vi "Read outside terminal.vi"(9 "FlatSequenceInnerTunnel in":refnum<class "FlatSequenceOuterTunnel.lvclass">) -> (3 "FlatSequenceInnerTunnel out":refnum<class "FlatSequenceOuterTunnel.lvclass">, 4 "outside terminal":refnum<class "Terminal.lvclass">)   [LabVIEW 2014, in "FlatSequenceOuterTunnel.lvclass"]
uses:
  FlatSequenceOuterTunnel.lvclass
  Terminal/Terminal.lvclass
  FlatSequenceOuterTunnel.lvclass/FlatSequenceOuterTunnel.ctl
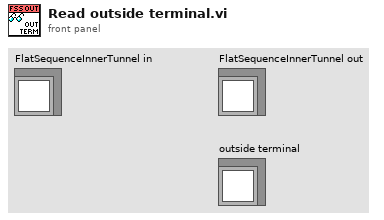
[diagram p1: front panel]
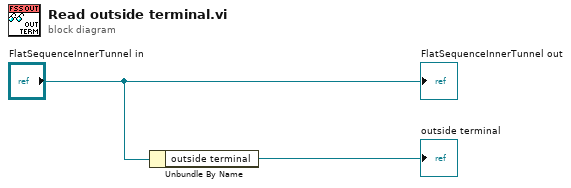
[diagram p0: block diagram]
diagram:
  n1 = Unbundle By Name("FlatSequenceInnerTunnel in") -> ("outside terminal"=→"outside terminal":refnum<class "Terminal.lvclass">)
  "FlatSequenceInnerTunnel out" <- "FlatSequenceInnerTunnel in"
